vi "448Issue2.vi"() -> ()   [LabVIEW 2017]
uses:
  user.lib/_NEVSTOP/Communicable State Machine(CSM)/Utility/_support/Periodic String Filter Level.ctl
  user.lib/_NEVSTOP/Communicable State Machine(CSM)/Utility/Periodic String Filter Setting.ctl
  user.lib/_NEVSTOP/Communicable State Machine(CSM)/Communicable State Machine.lvlib
  user.lib/_NEVSTOP/Communicable State Machine(CSM)/addons/Watchdog/CSM Watchdog.lvlib
  user.lib/_NEVSTOP/Communicable State Machine(CSM)/addons/Logger/CSM File Logger.lvlib
  user.lib/_NEVSTOP/Communicable State Machine(CSM)/addons/Logger/CSM File Logger Limit.ctl
panel:
  out "Waveform Chart":dbl(graph)
  out "Since Exiting(s)":dbl format="%.2f"
  out "LogInQ":i32
  out "State History":string
  out "log handling Speed(#/s)":dbl
  out "LogInQ changing Speed(#/s)":dbl
  out "Level":T1
  out "Module Names":string[](array[string])
  in  "Exit Modules":bool
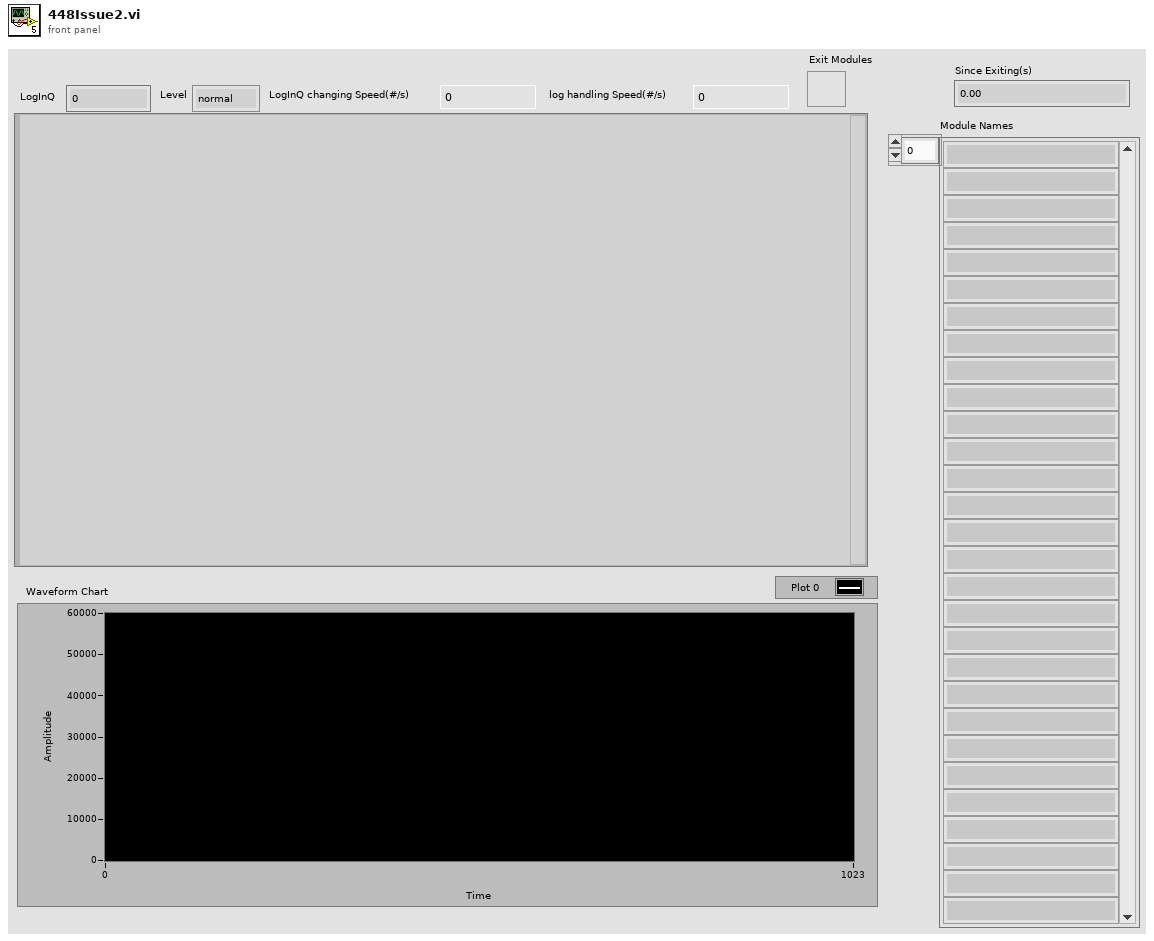
[diagram p1: front panel]
types:
  T1 = typedef "Communicable State Machine.lvlib/Periodic String Filter Level.ctl" = enum16{"normal", "L1", "L2", "L3", "L4"}
  T2 = typedef "CSM File Logger.lvlib/CSM File Logger Limit.ctl" = cluster{"file size (in bytes)":i64, "file num":i32}
  T3 = typedef "Communicable State Machine.lvlib/Periodic String Filter Setting.ctl" = cluster{"threashold(#/s)":dbl, "Check Peroid(s)":dbl}
  T4 = typedef "Communicable State Machine.lvlib/_CSM_GlobalLog_MSG.ctl" = cluster{"Name(\"\" to use uuid)":string, "Current State":string, "Arguments":string, "Source Message":T5, "Source Module":string, "Complete(T)/Start(F)":bool, "LogType":T6, "Time Stamp":timestamp}
  T5 = typedef "Communicable State Machine.lvlib/_CSM_Response Source Message.ctl" = cluster{"‘State":string, "’Arguments":string, "’Error":errorcluster}
  T6 = typedef "Communicable State Machine.lvlib/_CSM_GlobalLog_MSG_TYPE.ctl" = enum16{"User Log", "State Change", "Status", "Interrupt", "Register", "Unregister", "Error Log", "Module Created", "Module Destroyed"}
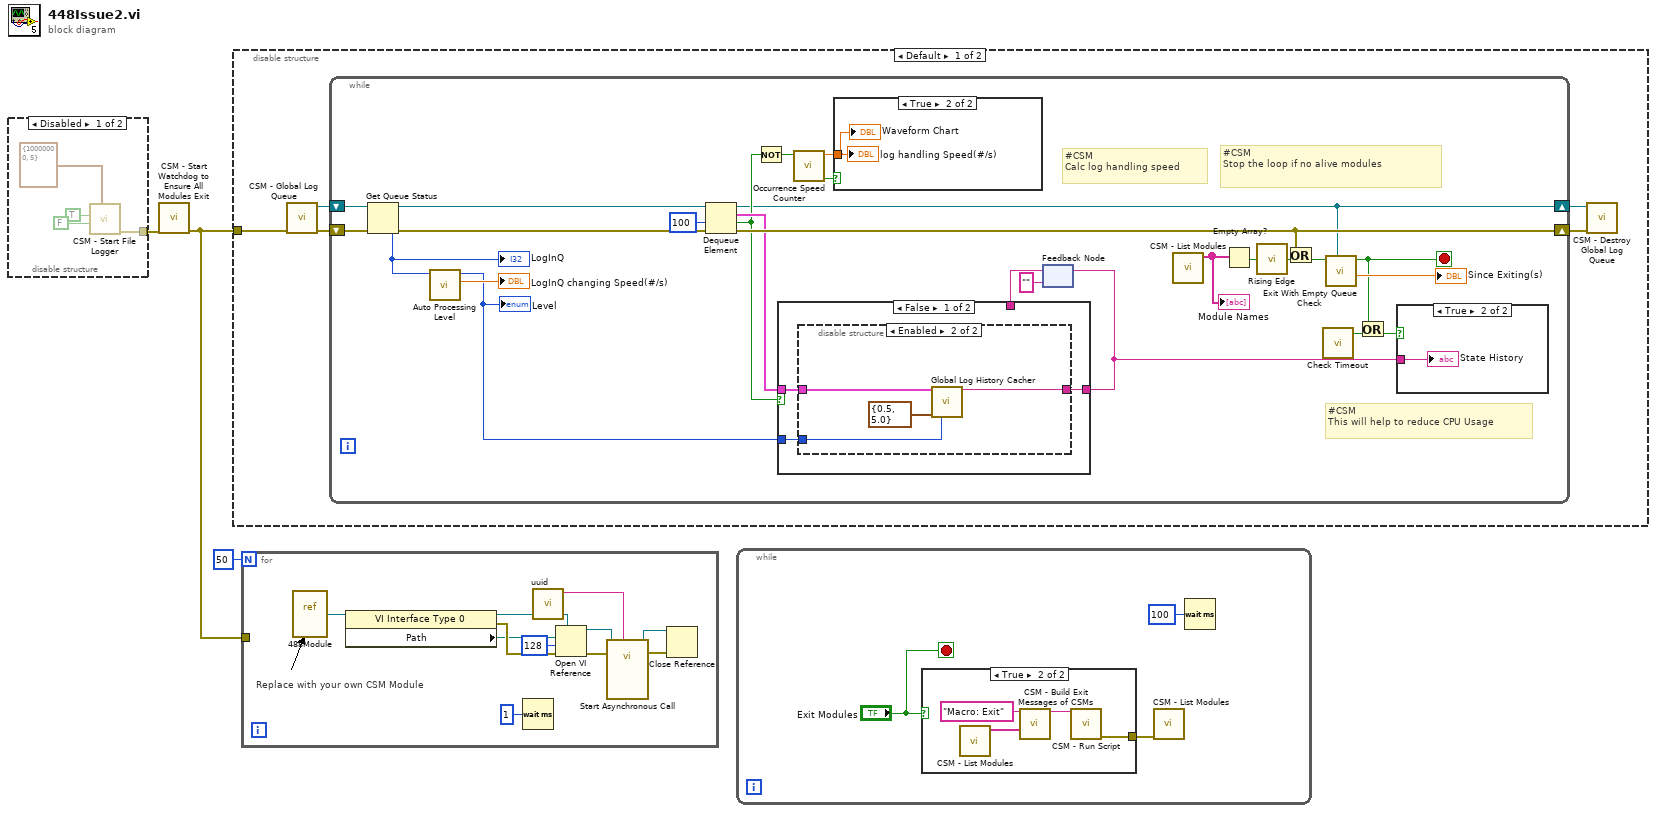
[diagram p0: block diagram]
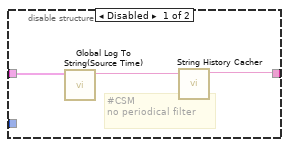
[diagram p3: hidden frame]
diagram:
  n1 = disable-structure shown="Disabled" {
    disable-tunnel: [w7 _] -> w2
    frame Disabled {
      n2 = call "CSM - Start File Logger.vi"("log limit"=T2 {"file size (in bytes)"=10000000, "file num"=5}, "WatchDog? (T)"=FALSE, "Exit When All Module Exist?(F)"=TRUE) -> ("Error out"=w7:errorcluster)  [unwired: 6 in, 2 out]
    }
    frame Enabled {
    }
  }
  n3 = call "CSM - Start Watchdog to Ensure All Modules Exit.vi"("error in (no error)"=w2) -> ("error out"=w1:errorcluster)  [unwired: 10 in]
  n4 = disable-structure shown="Default" {
    disable-tunnel: w1 -> [w8 _]
    frame condition #0 (active) {
      n5 = call "CSM - Global Log Queue.vi"("Error in"=w8) -> ("Error out"=w11:errorcluster, "GlobalEvent Queue"=w9:refnum<queue>)  [unwired: 9 in]
      n6 = while {
        shift-right: [w37] -> w12
        shift-left: w11 -> [w34]
        shift-right: [w25] -> w10
        shift-left: w9 -> [w38]
        stop <- w17 stop-if-true
        # "#CSM\nCalc log handling speed"
        # "#CSM\nStop the loop if no alive modules"
        # "#CSM\nThis will help to reduce CPU Usage"
        n7 = Get Queue Status(queue=w38, error in (no error)=w34) -> (queue out=w36:refnum<queue>, error out=w35:errorcluster, # elements in queue=w21:i32)  [unwired: 1 in, 5 out]
        "LogInQ" <- w21
        n8 = call "Auto Processing Level.vi"("#Left In Q"=w21) -> ("LogInQ changing Speed(#/s)"=→"LogInQ changing Speed(#/s)":dbl, "Level"=w20:T1)  [unwired: 8 in, 1 out]
        "Level" <- w20
        n9 = Dequeue Element(queue=w36, timeout in ms (-1)=100, error in (no error)=w35) -> (queue out=w25:refnum<queue>, element=w33:T4, timed out?=w27:bool, error out=w37:errorcluster)
        n10 = Not(x=w27) -> (.not. x?=w26:bool)
        n11 = call "Occurrence Speed Counter.vi"("Occured?(T)"=w26) -> ("New?"=w15:bool, "Speed(#/s)"=w16:dbl)  [unwired: 8 in, 1 out]
        n12 = case shown="True" w15 {
          tunnel: w16 -> [_ w39]
          frame False {
          }
          frame True {
            "log handling Speed(#/s)" <- w39
            "Waveform Chart" <- w39
          }
        }
        n13 = feedback #1("" ("String Cache")) -> (w29:string)
        n14 = case shown="False" w27 {
          tunnel: w33 -> [w42 _]
          tunnel: [w41 w50] -> w30
          tunnel: w29 -> [_ w50]
          tunnel: w20 -> [w40 _]
          frame False {
            n15 = disable-structure shown="Enabled" {
              disable-tunnel: w42 -> [w45 w48]
              disable-tunnel: [w43 w49] -> w41
              disable-tunnel: w40 -> [_ w47]
              frame Disabled {
                # "#CSM \nno periodical filter"
                n16 = call "Global Log To String(Source Time).vi"("Log"=w45) -> ("Log String"=w44:string)  [unwired: 9 in]
                n17 = call "String History Cacher.vi"("String"=w44) -> ("String Cache"=w43:string)  [unwired: 10 in]
              }
              frame Enabled {
                n18 = call "Global Log History Cacher.vi"("Cross CSM Data"=w48, "Settings"=T3 {"threashold(#/s)"=0.5, "Check Peroid(s)"=5.0}, "Level(Normal)"=w47) -> ("String Cache"=w49:string)  [unwired: 11 in, 1 out]
              }
            }
          }
          frame True {
          }
        }
        n19 = feedback-in #1(w30) -> ()
        n20 = call "CSM - List Modules.vi"() -> ("Module Names"=w18:string[])  [unwired: 10 in, 1 out]
        "Module Names" <- w18
        n21 = Empty Array?(array=w18) -> (empty?=w14:bool)
        n22 = call "Rising Edge.vi"("signal"=w14) -> ("rising edge"=w13:bool)
        n23 = Or(x=w37, y=w13) -> (x .or. y?=w23:bool)
        n24 = call "Check Timeout.vi"() -> ("Timeout"=w31:bool)  [unwired: 8 in]
        n25 = call "Exit With Empty Queue Check.vi"("queue"=w25, "Stop"=w23) -> ("Since Exiting(s)"=→"Since Exiting(s)":dbl, "exit"=w17:bool)  [unwired: 8 in]
        n26 = Or(x=w17, y=w31) -> (x .or. y?=w24:bool)
        n27 = case shown="True" w24 {
          tunnel: w30 -> [_ w51]
          frame False {
          }
          frame True {
            "State History" <- w51
          }
        }
      }
      n28 = call "CSM - Destroy Global Log Queue.vi"("Error in"=w12, "CreatedQueue"=w10) -> ()  [unwired: 9 in, 1 out]
    }
    frame condition #1 {
    }
  }
  n29 = for {
    N: 50 -> [_]
    tunnel: w1 -> [_]
    # "Replace with your own CSM Module"
    n30 = vi-ref "488Module.vi"() -> (w55:refnum<vi>)
    n31 = property class="VI Interface Type 0"(reference=w55) -> (reference out=w59:refnum<vi>, error out=w57:errorcluster, "Path"=w56:path)  [unwired: 1 in]
    n32 = Wait (ms)(milliseconds to wait=u32 1) -> ()  [unwired: 1 out]
    n33 = call "uuid.vi"() -> ("UUID"=w53:string)  [unwired: 11 in]
    n34 = Open VI Reference(type specifier VI Refnum (for type only)=w59, vi path=w56, options=128, error in (no error)=w57) -> (vi reference=w58:refnum<vi>, error out=w54:errorcluster)  [unwired: 2 in]
    n35 = call-by-ref "Start Asynchronous Call"(reference=w58, error in=w54, "Name(\"\" to use uuid)"=w53) -> (reference out=w61:refnum<vi>, error out=w60:errorcluster)  [unwired: 11 in]
    n36 = Close Reference(reference=w61, error in (no error)=w60) -> ()  [unwired: 1 out]
  }
  n37 = while {
    stop <- "Exit Modules" stop-if-true
    n38 = case shown="True" "Exit Modules" {
      tunnel: [_ w67] -> w64
      frame False {
      }
      frame True {
        n39 = call "CSM - List Modules.vi"() -> ("Module Names"=w69:string[])  [unwired: 10 in, 1 out]
        n40 = call "CSM - Build Exit Messages of CSMs.vi"("State with Arguments(\"Macro: Exit“)"="Macro: Exit" ("State with Arguments(\"Macro: Exit“)"), "CSMs"=w69) -> ("States"=w66:string)  [unwired: 13 in]
        n41 = call "CSM - Run Script.vi"("CSM Scripts"=w66) -> ("error out"=w67:errorcluster)  [unwired: 12 in, 2 out]
      }
    }
    n42 = call "CSM - List Modules.vi"("Error in"=w64) -> ()  [unwired: 9 in, 2 out]
    n43 = Wait (ms)(milliseconds to wait=u32 100) -> ()  [unwired: 1 out]
  }
